vi "Send SessionDisconnectMessage.vi"(11 "SessionMailbox":refnum<queue>) -> (0 "error out":errorcluster)   [LabVIEW 2013, in "MQTT Server.lvlib" / "Server.lvclass"]
uses:
  Server.lvclass
  Response -- cluster.ctl
  Control Packets/ControlPacket/ControlPacket.lvclass
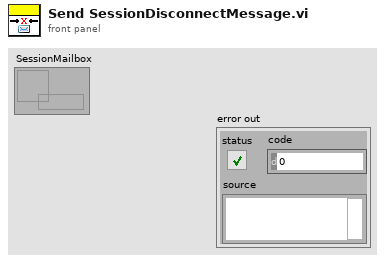
[diagram p1: front panel]
types:
  T1 = typedef "MQTT Server.lvlib/Server.lvclass/Response -- cluster.ctl" = cluster{"ServerResponse":refnum<class "ControlPacket.lvclass">, "Protocol Error":errorcluster, "disconnect":bool}
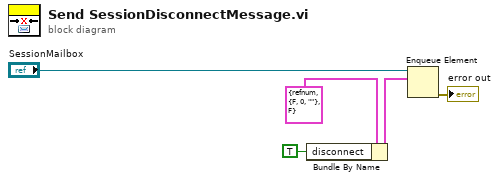
[diagram p0: block diagram]
diagram:
  n1 = Bundle By Name(cluster=T1 {"ServerResponse"=refnum, "Protocol Error"={"status"=FALSE, "code"=0, "source"=""}, "disconnect"=FALSE} ("Response"), "disconnect"=TRUE) -> (w3:T1)
  n2 = Enqueue Element(queue="SessionMailbox", element=w3) -> (error out=→"error out":errorcluster)  [unwired: 2 in, 2 out]
